vi "VisualizeNHRDC.vi"() -> ()   [LabVIEW 2018, in "Visualization.lvlib" / "VisualizeAcPwr.lvclass"]
uses:
  VisualizeAcPwr.lvclass
  VisualizeBase/VisualizeBase_class/Requests/clUserEventType.ctl
  <vilib>/event_ctls.llb/usereventprio.ctl
  AcPwr/AcPwrShared/clMeasurmentData.ctl
  <vilib>/Analysis/baseanly.llb/Mean (DBL).vi
  <vilib>/Utility/error.llb/Error Cluster From Error Code.vi
  <vilib>/ErrorRing/Error Ring.xnode
  VisualizeBase/VisualizeBase_class/VisualizeBase.lvclass
  <userlib>/NIST/NISTErrorLib/NISTErrorLib.lvlib
  <vilib>/Analysis/NI_AALBase.lvlib
  AcPwr/AcPwrShared/AcPwrShared.lvlib
panel:
  in  "Tab Control":enum32{"Chart", "XY Graph"}(tab)
  out "NHRDC":waveform(dbl)[](graph)=[{"t0"=timestamp(3657200531.6397257 s since 1904-01-01), "dt"=1.0, "Y"=[46.19]}, {"t0"=timestamp(3657200531.6397257 s since 1904-01-01), "dt"=1.0, "Y"=[2.0]}, {"t0"=timestamp(3657200531.6397257 s since 1904-01-01), "dt"=1.0, "Y"=[60.0]}]
  in  "PlotYAxis":u32[](array[numeric])=[0, 1, 0] max=1
  out "Incorrect DataType?":bool
  out "Current (A)":dbl(knob) scale=0.0..15.0
  out "Voltage (V)":dbl(knob) scale=0.0..100.0
  out "XY Graph":cluster{"Current":dbl[], "Voltage":dbl[]}[](graph)
  in  "Clear Graph":bool
  in  "PluginName":string="AcPwr.NHRDC0"
  out "ErrorArray":errorcluster[](array[cluster])
  in  "QueuName":string="NHRDCVQ"
  in  "btnStop":bool
  in  "btnReset":bool
  in  "btnClear":bool
  # "0=Left Axis and 1=Right Axis"
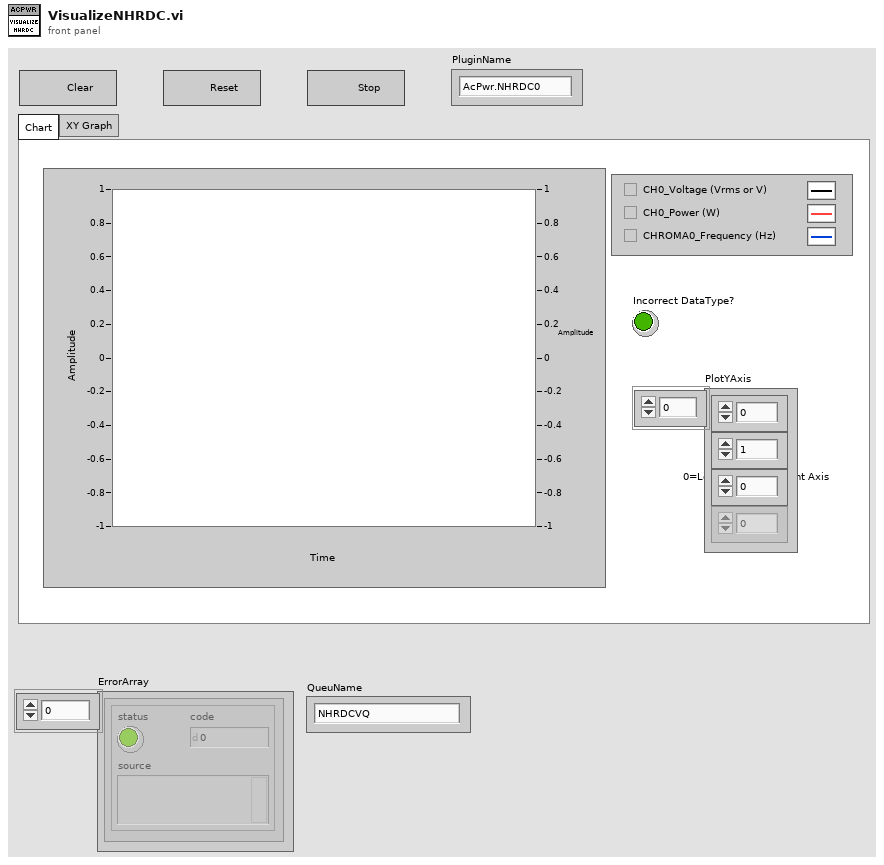
[diagram p1: front panel]
types:
  T1 = typedef "Visualization.lvlib/VisualizeBase.lvclass/clRequestEvents.ctl" = cluster{"StopRequest":refnum<user-event>, "ResetRequest":refnum<user-event>}
  T2 = typedef "AcPwrShared.lvlib/clBroadcastEvents.ctl" = cluster{"DidInit":refnum<user-event>, "StatusUpdate":refnum<user-event>, "ErrorReport":refnum<user-event>, "DidStop":refnum<user-event>, "PathToINI":refnum<user-event>, "Measurements":refnum<user-event>, "LoadConfigFile":refnum<user-event>, "GetSettings":refnum<user-event>, "SetSettings":refnum<user-event>, "GetType&ID":refnum<user-event>, "GotSettings":refnum<user-event>}
  T3 = typedef "usereventprio.ctl" = enum32{"high priority", "normal priority"}
  T4 = typedef "Visualization.lvlib/VisualizeBase.lvclass/clUserEventType.ctl" = cluster{"BusIndex":i8, "Data":variant}
  T5 = typedef "AcPwrShared.lvlib/clMeasurmentData.ctl" = cluster{"MeasName":string, "XML Data":string, "WaveformData":waveform(dbl)[]}
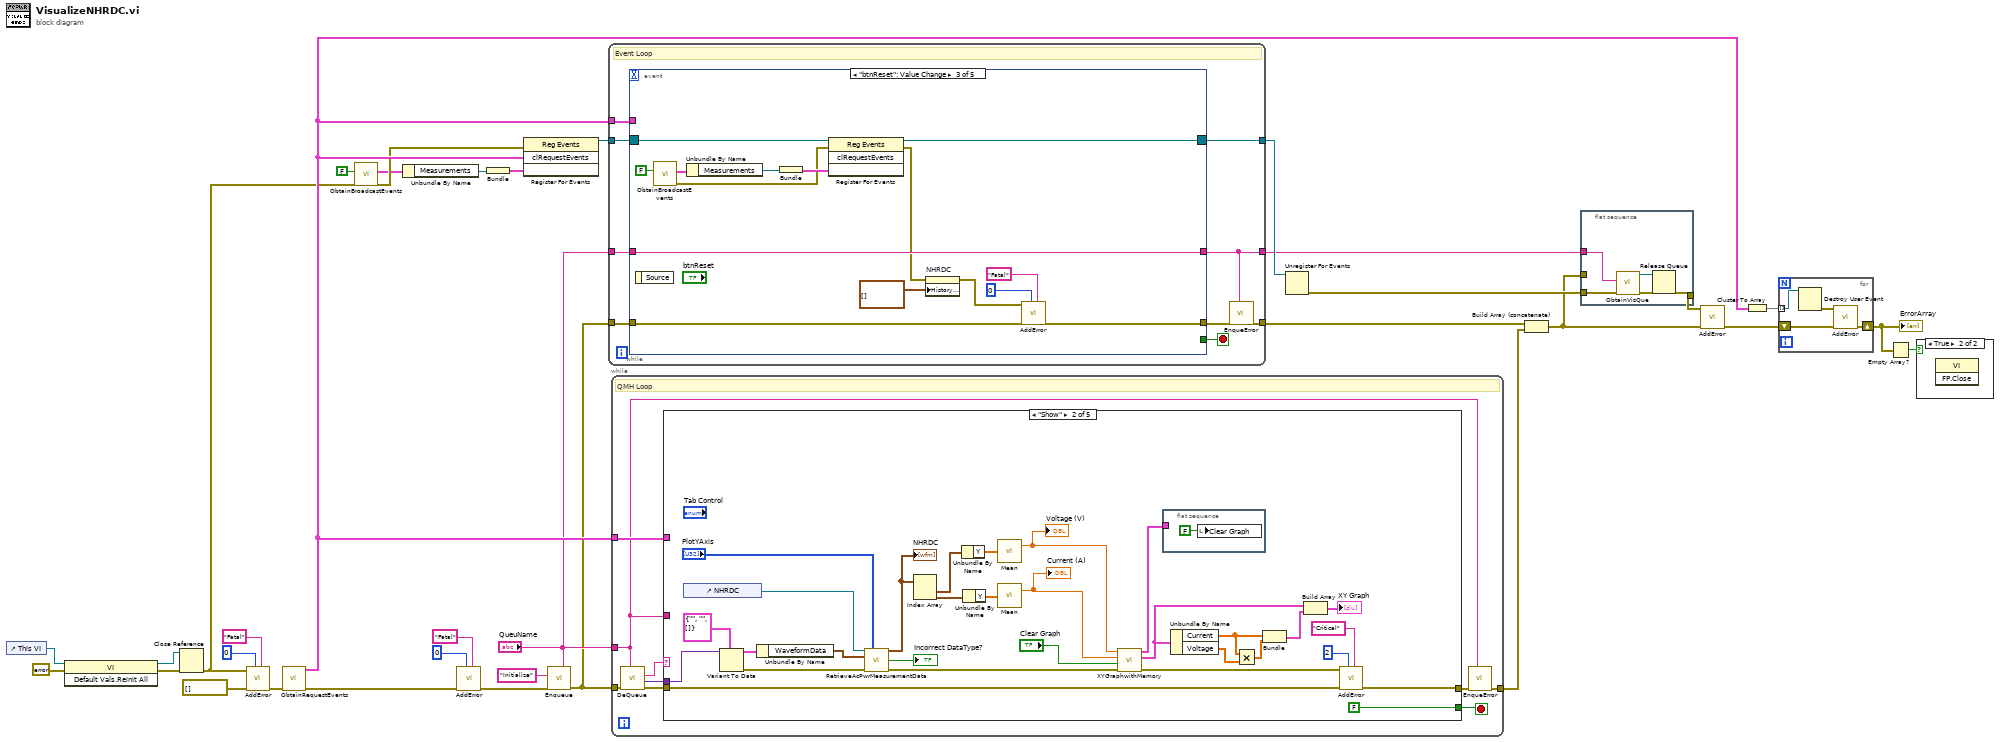
[diagram p0: block diagram]
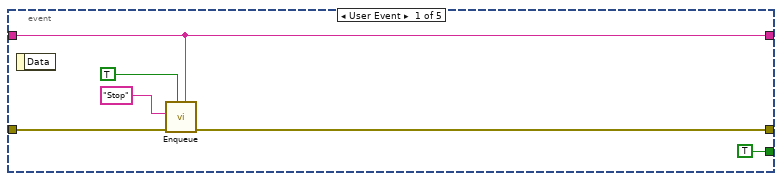
[diagram p2: hidden frame]
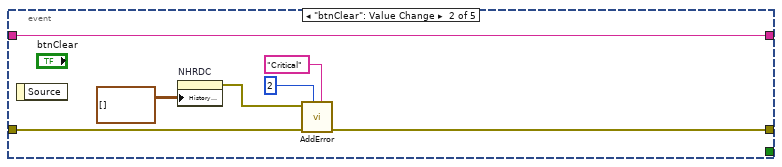
[diagram p3: hidden frame]
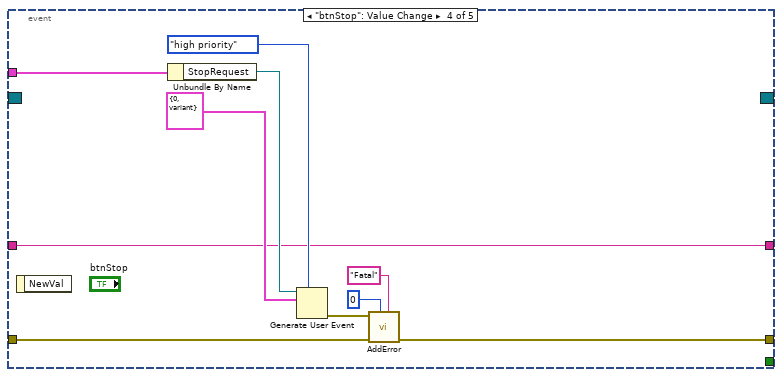
[diagram p4: hidden frame]
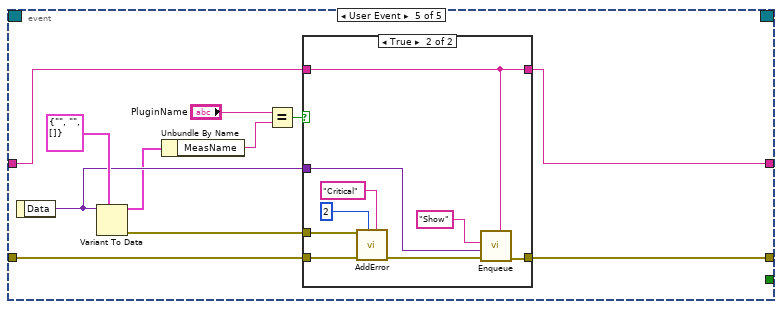
[diagram p5: hidden frame]
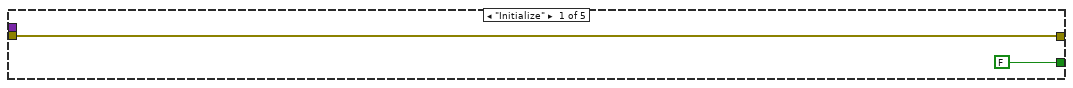
[diagram p7: hidden frame]
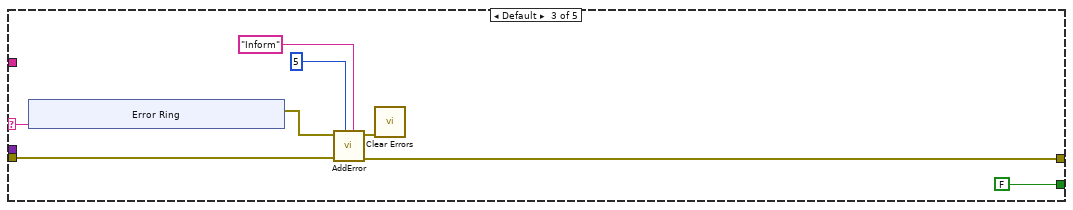
[diagram p8: hidden frame]
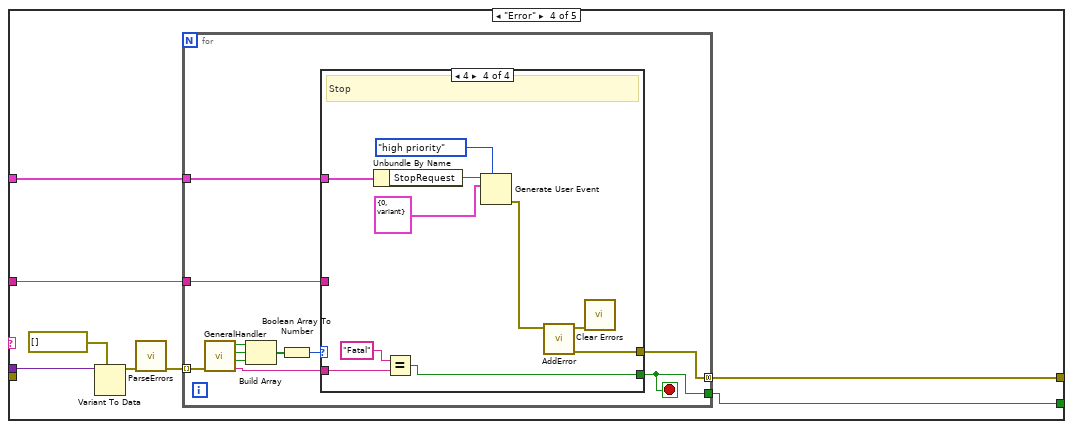
[diagram p9: hidden frame]
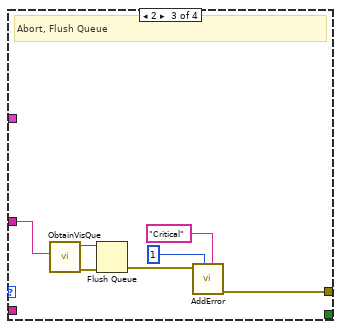
[diagram p12: hidden frame]
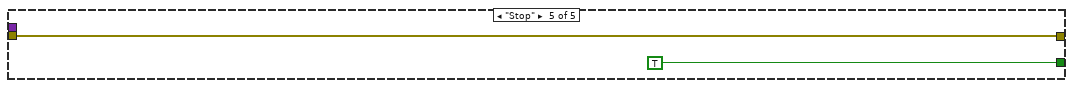
[diagram p13: hidden frame]
diagram:
  n1 = control-ref of="This VI"() -> (w20:refnum<vi>)
  n2 = invoke class="VI" method="Default Vals.Reinit All"(reference=w20, error in=errorcluster {"status"=FALSE, "code"=0, "source"=""} ("error in (no error)")) -> (reference out=w17:refnum<vi>, error out=w18:errorcluster)  [unwired: 1 in, 1 out]
  n3 = Close Reference(reference=w17, error in (no error)=w18) -> (error out=w15:errorcluster)
  n4 = call <userlib>:"AddError.vi"("Severity"="Fatal" ("String"), "Priority"=u8 0, "ErrorArray"=errorcluster[] [], "error in (no error)"=w15) -> ("ErrorArray"=w32:errorcluster[])  [unwired: 6 in, 1 out]
  n5 = call "ObtainRequestEvents.vi"("Error"=w32) -> ("Error"=w5:errorcluster[], "clRequestEvents"=w24:T1)  [unwired: 9 in]
  n6 = call "ObtainBroadcastEvents.vi"("error in (no error)"=w15, "CreateNew? (F)"=FALSE) -> ("error out"=w14:errorcluster, "clAcPwrEvents"=w13:T2)  [unwired: 8 in]
  n7 = Unbundle By Name(w13) -> ("Measurements"=w22:refnum<user-event>)
  n8 = call <userlib>:"AddError.vi"("Severity"="Fatal" ("String"), "Priority"=u8 0, "ErrorArray"=w5) -> ("ErrorArray"=w4:errorcluster[])  [unwired: 7 in, 1 out]
  n9 = Bundle("Measurements"=w22) -> (w21:cluster{"Measurements":refnum<user-event>})  [unwired: 1 in]
  n10 = register-events(error in=w14, w24, w21) -> (reference out=w33:refnum<event-registration>)  [unwired: 1 in, 1 out]
  n11 = call "Enqueue.vi"("QueName"="QueuName", "Error"=w4, "Message"="Initialize") -> ("Error"=w3:errorcluster[])  [unwired: 8 in]
  n12 = while {
    tunnel: w33 -> [w43]
    tunnel: [w40] -> w29
    tunnel: [w39] -> w31
    tunnel: w24 -> [w38]
    tunnel: w3 -> [w37]
    tunnel: "QueuName" -> [w36]
    tunnel: [w35] -> w11
    stop <- w42 stop-if-true
    # "Event Loop"
    n13 = event shown="[2] \"btnReset\": Value Change" {
      selector: w43 -> [_ _ w71 _ _]
      dyn-events: [_ _ w70 _ _] -> w39
      timeout: _ -> [_ _ _ _ _]
      tunnel: [TRUE _ _ _ _] -> w42
      tunnel: [w48 w53 w64 w79 w92] -> w41
      tunnel: w38 -> [_ _ _ w74 _]
      tunnel: w37 -> [w45 w52 w63 w72 w88]
      tunnel: w36 -> [w44 w56 w65 w73 w90]
      tunnel: [w44 w56 w65 w73 w89] -> w35
      event User Event {
        n14 = event-data() -> ()  [unwired: 1 in, 1 out]
        n15 = call "Enqueue.vi"("QueName"=w44, "Priority? (F)"=TRUE, "Error"=w45, "Message"="Stop") -> ("Error"=w48:errorcluster[])  [unwired: 7 in]
      }
      event "btnClear": Value Change {
        n16 = event-data() -> ()  [unwired: 1 in, 1 out]
        n17 = property on="NHRDC" class="WFChart (strict)"("History Data"=waveform(dbl)[][] []) -> (error out=w50:errorcluster)  [unwired: 2 in, 1 out]
        n18 = call <userlib>:"AddError.vi"("Severity"="Critical" ("String"), "Priority"=u8 2, "ErrorArray"=w52, "error in (no error)"=w50) -> ("ErrorArray"=w53:errorcluster[])  [unwired: 6 in, 1 out]
      }
      event "btnReset": Value Change {
        n19 = event-data() -> ()  [unwired: 1 in, 1 out]
        n20 = call "ObtainBroadcastEvents.vi"("CreateNew? (F)"=FALSE) -> ("error out"=w66:errorcluster, "clAcPwrEvents"=w67:T2)  [unwired: 9 in]
        n21 = Unbundle By Name(w67) -> ("Measurements"=w69:refnum<user-event>)
        n22 = Bundle("Measurements"=w69) -> (w68:cluster{"Measurements":refnum<user-event>})  [unwired: 1 in]
        n23 = register-events(reference=w71, error in=w66, w68) -> (reference out=w70:refnum<event-registration>, error out=w59:errorcluster)  [unwired: 1 in]
        n24 = property on="NHRDC" class="WFChart (strict)"(error in=w59, "History Data"=waveform(dbl)[][] []) -> (error out=w60:errorcluster)  [unwired: 1 in, 1 out]
        n25 = call <userlib>:"AddError.vi"("Severity"="Fatal" ("String"), "Priority"=u8 0, "ErrorArray"=w63, "error in (no error)"=w60) -> ("ErrorArray"=w64:errorcluster[])  [unwired: 6 in, 1 out]
      }
      event "btnStop": Value Change {
        n26 = event-data() -> ()  [unwired: 1 in, 1 out]
        n27 = Unbundle By Name(w74) -> ("StopRequest"=w80:refnum<user-event>)
        n28 = Generate User Event(priority (normal)=usereventprio."high priority", user event=w80, event data cluster=T4 {"BusIndex"=0, "Data"=variant} ("event data")) -> (error out=w81:errorcluster)  [unwired: 1 in, 1 out]
        n29 = call <userlib>:"AddError.vi"("Severity"="Fatal" ("String"), "Priority"=u8 0, "ErrorArray"=w72, "error in (no error)"=w81) -> ("ErrorArray"=w79:errorcluster[])  [unwired: 6 in, 1 out]
      }
      event User Event {
        n30 = event-data() -> ("Data"=w84:variant)  [unwired: 1 in]
        n31 = Variant To Data(type=T5 {"MeasName"="", "XML Data"="", "WaveformData"=[]} ("MeasurmentDataCluster"), Variant=w84) -> (data=w83:T5, error out=w87:errorcluster)  [unwired: 1 in]
        n32 = Unbundle By Name(w83) -> ("MeasName"=w82:string)
        n33 = Equal?(x="PluginName", y=w82) -> (x = y?=w91:bool)
        n34 = case shown="True" w91 {
          tunnel: [w94 w102] -> w92
          tunnel: w88 -> [w94 w97]
          tunnel: w90 -> [w93 w101]
          tunnel: [w93 w101] -> w89
          tunnel: w84 -> [_ w100]
          tunnel: w87 -> [_ w95]
          frame False {
          }
          frame True {
            n35 = call <userlib>:"AddError.vi"("Severity"="Critical" ("String"), "Priority"=u8 2, "ErrorArray"=w97, "error in (no error)"=w95) -> ("ErrorArray"=w96:errorcluster[])  [unwired: 6 in, 1 out]
            n36 = call "Enqueue.vi"("QueName"=w101, "Error"=w96, "Data"=w100, "Message"="Show") -> ("Error"=w102:errorcluster[])  [unwired: 7 in]
          }
        }
      }
    }
    n37 = call "EnqueError.vi"("QueName"=w35, "Error"=w41) -> ("Error"=w40:errorcluster[])  [unwired: 9 in]
  }
  n38 = while {
    tunnel: w3 -> [w112]
    tunnel: [w106] -> w28
    tunnel: "QueuName" -> [w104]
    tunnel: w24 -> [w105]
    stop <- w107 stop-if-true
    # "QMH Loop"
    n39 = call "DeQueue.vi"("QueName"=w104, "Error"=w112) -> ("Error"=w109:errorcluster[], "Data"=w110:variant, "Message"=w111:string)  [unwired: 7 in]
    n40 = case shown="\"Show\"" w111 {
      selector: w111 -> [_ _ w153 _ _]
      tunnel: w110 -> [_ w140 _ w168 _]
      tunnel: w109 -> [w114 w141 w151 _ w197]
      tunnel: [w114 w144 w150 w164 w197] -> w108
      tunnel: [FALSE FALSE FALSE w163 TRUE] -> w107
      tunnel: w105 -> [_ _ _ w162 _]
      tunnel: w104 -> [_ _ _ w161 _]
      frame "Initialize" {
      }
      frame "Show" {
        n41 = control-ref of="NHRDC"() -> (w115:refnum<vi>)
        n42 = Variant To Data(type=T5 {"MeasName"="", "XML Data"="", "WaveformData"=[]} ("MeasurmentDataCluster"), Variant=w140) -> (data=w119:T5, error out=w122:errorcluster)  [unwired: 1 in]
        n43 = Unbundle By Name(w119) -> ("WaveformData"=w118:waveform(dbl)[])
        n44 = call "RetrieveAcPwrMeasurementData.vi"("WaveformChartReference"=w115, "PlotYScale"="PlotYAxis", "WaveformArrayIn"=w118, "error in (no error)"=w122) -> ("WaveformArrayOut"=w116:waveform(dbl)[], "Incorrect DataType?"=→"Incorrect DataType?":bool, "error out"=w121:errorcluster)  [unwired: 7 in, 2 out]
        "NHRDC" <- w116
        n45 = Index Array(array=w116) -> (element #1=w139:waveform(dbl), element #2=w138:waveform(dbl))  [unwired: 2 in]
        n46 = Unbundle By Name(w139) -> ("Y"=w136:dbl[])
        n47 = Unbundle By Name(w138) -> ("Y"=w135:dbl[])
        n48 = call-poly <vilib>:"Mean.vi"("X"=w136) -> ("mean"=w133:dbl)  [unwired: 1 out]
        "Voltage (V)" <- w133
        n49 = call-poly <vilib>:"Mean.vi"("X"=w135) -> ("mean"=w131:dbl)  [unwired: 1 out]
        "Current (A)" <- w131
        n50 = call "XYGraphwithMemory.vi"("Error In"=w121, "Clear Graph"="Clear Graph", "Current"=w131, "Voltage"=w133) -> ("Error Out"=w132:errorcluster, "output cluster"=w129:cluster{"Current":dbl[], "Voltage":dbl[]}, "Cluster"=w130:cluster{"Array":dbl[], "Array":dbl[]})  [unwired: 5 in]
        n51 = flat-sequence {
          tunnel: w130 -> [_]
          frame #0 {
            n52 = local write "Clear Graph"(FALSE ("Clear Graph")) -> ()
          }
        }
        n53 = Unbundle By Name(w129) -> ("Current"=w125:dbl[], "Voltage"=w126:dbl[])
        n54 = Multiply(x=w125, y=w126) -> (x*y=w124:dbl[])
        n55 = Bundle("Current"=w125, w124) -> (w127:cluster{"Current":dbl[], dbl[]})  [unwired: 1 in]
        n56 = Build Array(w129, w127) -> (→"XY Graph":cluster{"Current":dbl[], "Voltage":dbl[]}[])
        n57 = call <userlib>:"AddError.vi"("Severity"="Critical" ("String"), "Priority"=u8 2, "ErrorArray"=w141, "error in (no error)"=w132) -> ("ErrorArray"=w144:errorcluster[])  [unwired: 6 in, 1 out]
      }
      frame Default {
        n58 = xnode "Error Ring"("parameter 0"=w153) -> ("error out"=w152:errorcluster)
        n59 = call <userlib>:"AddError.vi"("Severity"="Inform" ("String"), "Priority"=u8 5, "ErrorArray"=w151, "error in (no error)"=w152) -> ("ErrorArray"=w150:errorcluster[], "error out"=w149:errorcluster)  [unwired: 6 in]
        n60 = call <vilib>:"Clear Errors.vi"("error in (no error)"=w149) -> ()  [unwired: 5 in, 2 out]
      }
      frame "Error" {
        n61 = Variant To Data(type=errorcluster[] [], Variant=w168) -> (data=w166:errorcluster[])  [unwired: 1 in, 1 out]
        n62 = call <userlib>:"ParseErrors.vi"("ErrorArray"=w166) -> ("ErrorArray"=w165:errorcluster[])  [unwired: 8 in, 2 out]
        n63 = for {
          tunnel: w165 -> [w179] mode=indexing
          tunnel: [w173] -> w164 mode=concatenating
          tunnel: [w171] -> w163
          tunnel: w162 -> [w170]
          tunnel: w161 -> [w169]
          stop <- w171 stop-if-true
          n64 = call <userlib>:"GeneralHandler.vi"("error in (no error)"=w179) -> ("Severity"=w172:string, "Stop"=w176:bool, "Abort"=w177:bool, "Continue"=w178:bool)  [unwired: 7 in]
          n65 = Build Array(w178, w177, w176) -> (w175:bool[])
          n66 = Boolean Array To Number(Boolean array=w175) -> (number=w174:u32)
          n67 = case shown="4" w174 {
            tunnel: [_ _ w184 w195] -> w173
            tunnel: w172 -> [_ _ _ w190]
            tunnel: [_ _ _ w188] -> w171
            tunnel: w170 -> [_ _ _ w187]
            tunnel: w169 -> [_ _ w180 _]
            frame 0, Default {
              # "No Dialog"
            }
            frame 1 {
              # "Continue"
            }
            frame 2 {
              # "Abort, Flush Queue"
              n68 = call "ObtainVisQue.vi"("QueName"=w180) -> ("error out"=w186:errorcluster, "queue out"=w185:refnum<queue>)  [unwired: 9 in]
              n69 = Flush Queue(queue=w185, error in (no error)=w186) -> (error out=w183:errorcluster)  [unwired: 2 out]
              n70 = call <userlib>:"AddError.vi"("Severity"="Critical" ("String"), "Priority"=u8 1, "error in (no error)"=w183) -> ("ErrorArray"=w184:errorcluster[])  [unwired: 7 in, 1 out]
            }
            frame 4 {
              # "Stop"
              n71 = Unbundle By Name(w187) -> ("StopRequest"=w196:refnum<user-event>)
              n72 = Equal?(x="Fatal", y=w190) -> (x = y?=w188:bool)
              n73 = Generate User Event(priority (normal)=usereventprio."high priority", user event=w196, event data cluster=T4 {"BusIndex"=0, "Data"=variant} ("event data")) -> (error out=w194:errorcluster)  [unwired: 1 in, 1 out]
              n74 = call <userlib>:"AddError.vi"("error in (no error)"=w194) -> ("ErrorArray"=w195:errorcluster[], "error out"=w191:errorcluster)  [unwired: 9 in]
              n75 = call <vilib>:"Clear Errors.vi"("error in (no error)"=w191) -> ()  [unwired: 5 in, 2 out]
            }
          }
        }
      }
      frame "Stop" {
      }
    }
    n76 = call "EnqueError.vi"("QueName"=w104, "Error"=w108) -> ("Error"=w106:errorcluster[])  [unwired: 9 in]
  }
  n77 = Unregister For Events(event registration refnum=w31) -> (error out=w27:errorcluster)  [unwired: 1 in]
  n78 = Build Array (concatenate)(w29, w28) -> (w2:errorcluster[])
  n79 = flat-sequence {
    tunnel: w27 -> [w203]
    tunnel: [w200] -> w26
    tunnel: w11 -> [w199]
    tunnel: w2 -> [_]
    frame #0 {
      n80 = call "ObtainVisQue.vi"("error in (no error)"=w203, "QueName"=w199) -> ("error out"=w202:errorcluster, "queue out"=w201:refnum<queue>)  [unwired: 8 in]
      n81 = Release Queue(queue=w201, error in (no error)=w202) -> (error out=w200:errorcluster)  [unwired: 1 in, 2 out]
    }
  }
  n82 = call <userlib>:"AddError.vi"("ErrorArray"=w2, "error in (no error)"=w26) -> ("ErrorArray"=w25:errorcluster[])  [unwired: 8 in, 1 out]
  n83 = Cluster To Array(cluster=w24) -> (array=w30:refnum<user-event>[])
  n84 = for {
    tunnel: w30 -> [w207] mode=indexing
    shift-right: [w206] -> w16
    shift-left: w25 -> [w205]
    n85 = Destroy User Event(user event=w207) -> (error out=w204:errorcluster)  [unwired: 1 in]
    n86 = call <userlib>:"AddError.vi"("ErrorArray"=w205, "error in (no error)"=w204) -> ("ErrorArray"=w206:errorcluster[])  [unwired: 8 in, 1 out]
  }
  "ErrorArray" <- w16
  n87 = Empty Array?(array=w16) -> (empty?=w23:bool)
  n88 = case shown="True" w23 {
    frame False {
    }
    frame True {
      n89 = invoke class="VI" method="FP.Close"() -> ()  [unwired: 3 in, 3 out]
    }
  }
